vi "etlWriteFuncGenWithDelayedSignal.vi"(1 "max (dpt)":dbl, 2 "min (dpt)":dbl, 3 "minmax":bool) -> ()   [LabVIEW 2017]
uses:
  <vilib>/DAQmx/write.llb/DAQmx Write (Analog 2D DBL NChan NSamp).vi
  globalDevices.vi
  globalUtilities.vi
  <vilib>/DAQmx/miscellaneous.llb/DAQmx Fill In Error Info.vi
panel:
  out "max step":dbl
  out "success":bool
  out "Waveform Graph 3":dbl[][](graph)
  out "nT":i32
  out "dt":dbl
  out "omega":dbl
  out "amplitude":dbl
  out "offset":dbl
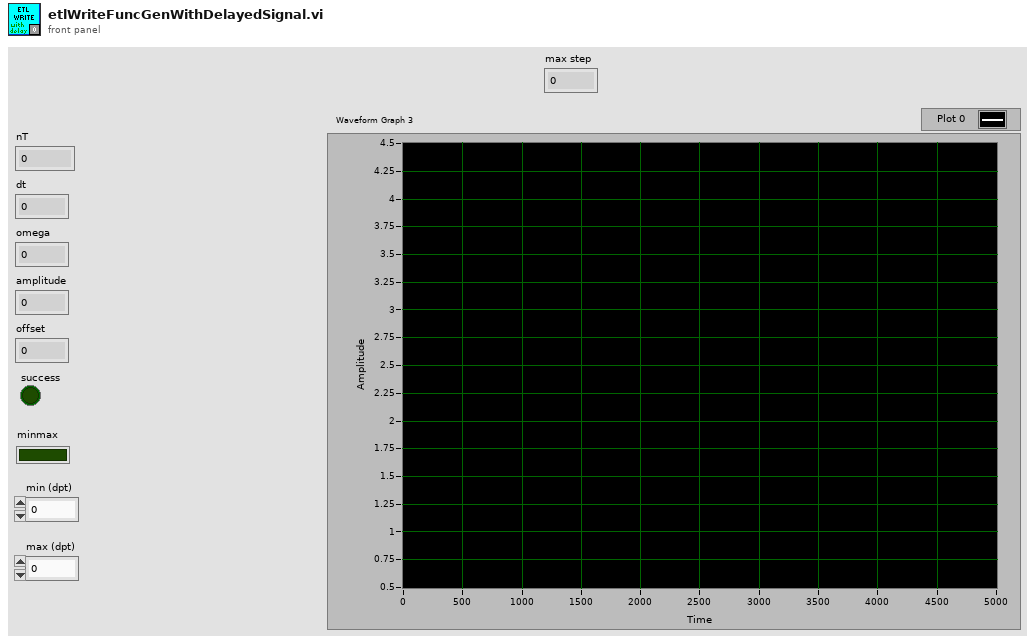
[diagram p1: front panel]
types:
  T1 = cluster{"waveform":dbl[], "latencyShiftPermutation":i32, "V/um":dbl, "waveType":string, "etlCalibrationMindpt":dbl, "etlCalibrationMaxdpt":dbl, "piezoEtlClockLock":bool, "volumeHeight":dbl, "volumeHeightUnits":string, "etl dpt/um":dbl, "etlVMin":dbl, "etlVMax":dbl}
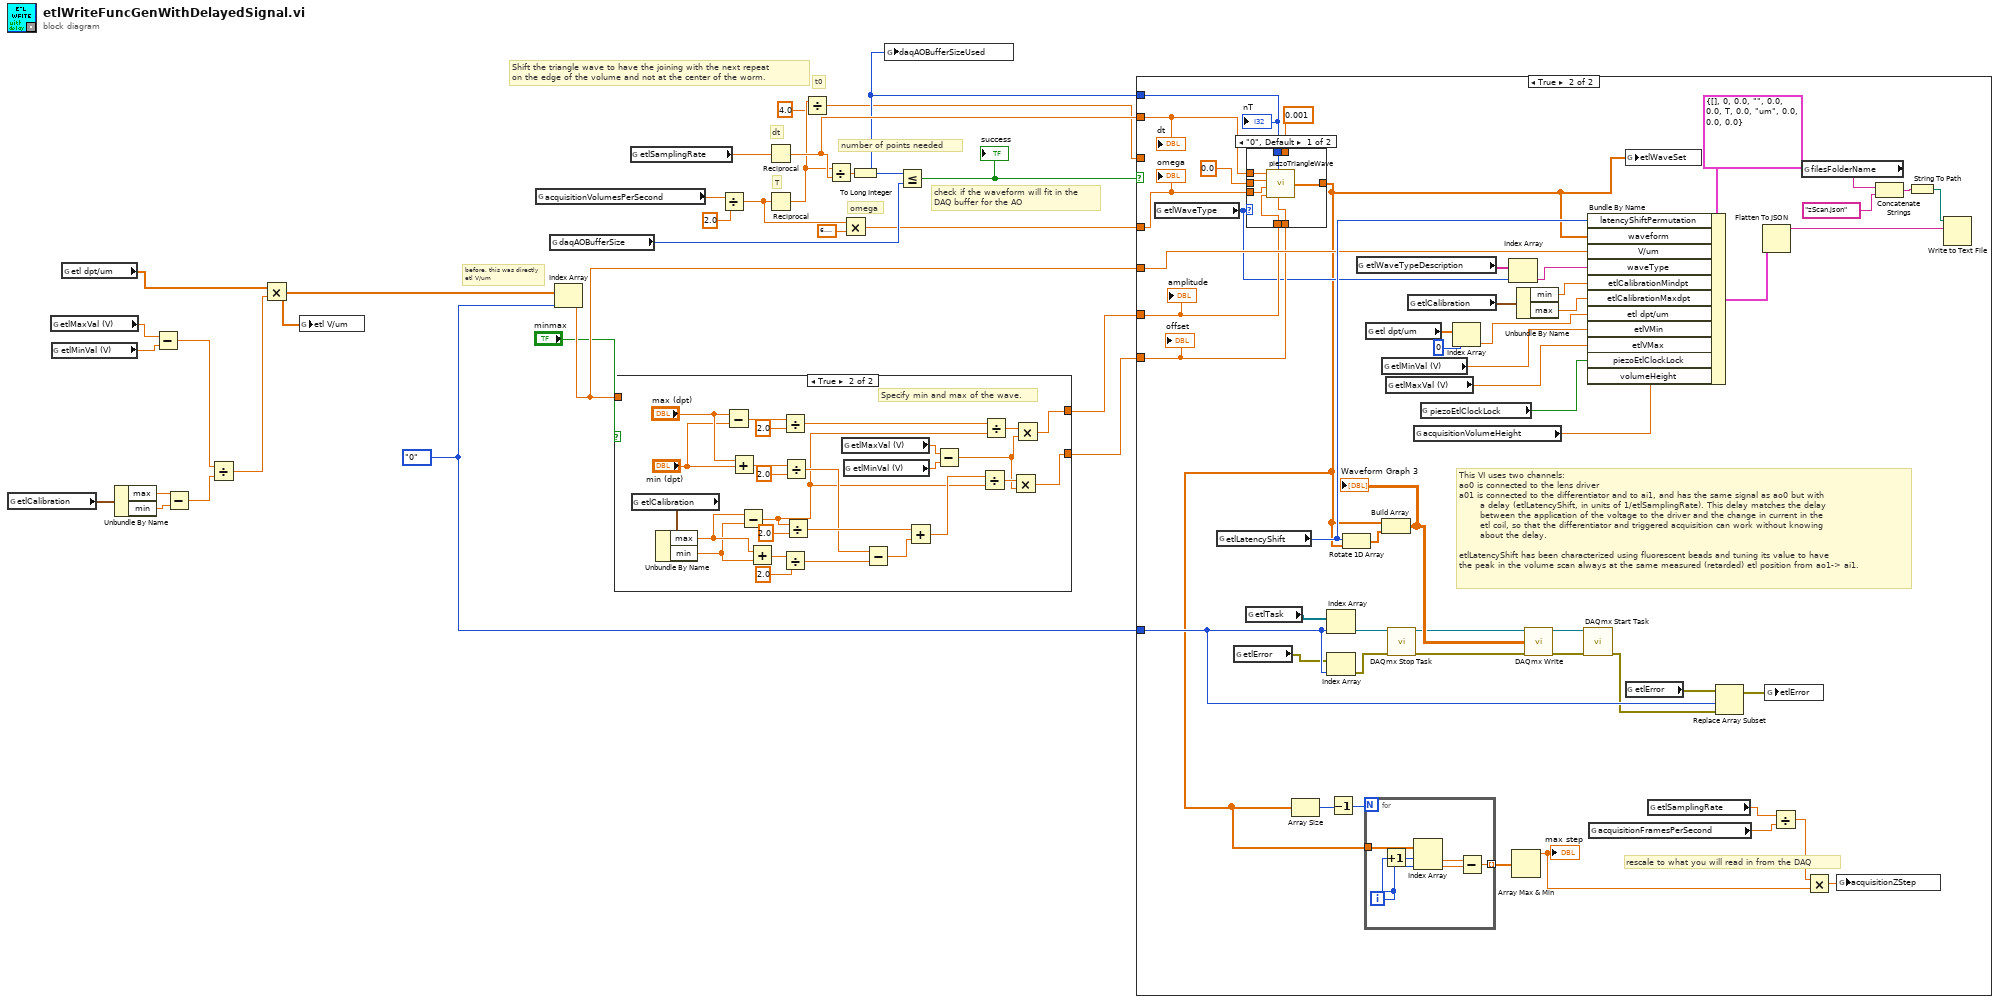
[diagram p0: block diagram]
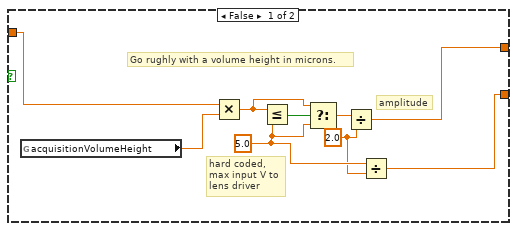
[diagram p2: hidden frame]
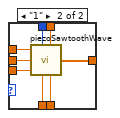
[diagram p4: hidden frame]
diagram:
  w17 = enum16{"0", "1"}."0" ("lens")
  # "Shift the triangle wave to have the joining with the next repeat\non the edge of the volume and not at the center of the worm."
  # "t0"
  # "before, this was directly\netl V/um"
  # "check if the waveform will fit in the\nDAQ buffer for the AO"
  # "omega"
  # "number of points needed"
  # "T"
  # "dt"
  n1 = global read "globalDevices.vi" "etlCalibration"() -> (w14:cluster{"min":dbl, "max":dbl})
  n2 = global read "globalDevices.vi" "etlMaxVal (V)"() -> (w11:dbl)
  n3 = global read "globalDevices.vi" "etlMinVal (V)"() -> (w10:dbl)
  n4 = global read "globalDevices.vi" "etl dpt/um"() -> (w7:dbl[])
  n5 = Unbundle By Name(w14) -> ("max"=w13:dbl, "min"=w12:dbl)
  n6 = Subtract(x=w11, y=w10) -> (x-y=w9:dbl)
  n7 = Subtract(x=w13, y=w12) -> (x-y=w8:dbl)
  n8 = Divide(x=w9, y=w8) -> (x/y=w6:dbl)
  n9 = Multiply(x=w7, y=w6) -> (x*y=w5:dbl[])
  n10 = global write "globalDevices.vi" "etl V/um"(w5) -> ()
  n11 = global read "globalUtilities.vi" "acquisitionVolumesPerSecond"() -> (w28:dbl)
  n12 = global read "globalDevices.vi" "daqAOBufferSize"() -> (w26:i32)
  n13 = Index Array(array=w5, index=w17) -> (element=w16:dbl)
  n14 = case shown="True" "minmax" {
    tunnel: [w34 w51] -> w25
    tunnel: [w31 w39] -> w18
    tunnel: w16 -> [w30 _]
    frame False {
      w33 = 5.0 ("y")
      w32 = 2.0 ("y")
      # "Go rughly with a volume height in microns."
      # "hard coded,\nmax input V to\nlens driver"
      # "amplitude"
      n15 = global read "globalUtilities.vi" "acquisitionVolumeHeight"() -> (w38:dbl)
      n16 = Multiply(x=w30, y=w38) -> (x*y=w36:dbl)
      n17 = Less Or Equal?(x=w36, y=w33) -> (x <= y?=w37:bool)
      n18 = Select(t=w36, s=w37, f=w33) -> (s? t:f=w35:dbl)
      n19 = Divide(x=w35, y=w32) -> (x/y=w34:dbl)
      n20 = Divide(x=w33, y=w32) -> (x/y=w31:dbl)
    }
    frame True {
      # "Specify min and max of the wave."
      n21 = global read "globalDevices.vi" "etlCalibration"() -> (w58:cluster{"min":dbl, "max":dbl})
      n22 = Unbundle By Name(w58) -> ("max"=w57:dbl, "min"=w56:dbl)
      n23 = Subtract(x="max (dpt)", y="min (dpt)") -> (x-y=w64:dbl)
      n24 = Add(x="max (dpt)", y="min (dpt)") -> (x+y=w59:dbl)
      n25 = Subtract(x=w57, y=w56) -> (x-y=w40:dbl)
      n26 = Add(x=w57, y=w56) -> (x+y=w55:dbl)
      n27 = Divide(x=w64, y=2.0) -> (x/y=w53:dbl)
      n28 = Divide(x=w55, y=2.0) -> (x/y=w47:dbl)
      n29 = Divide(x=w59, y=2.0) -> (x/y=w48:dbl)
      n30 = Divide(x=w40, y=2.0) -> (x/y=w49:dbl)
      n31 = global read "globalDevices.vi" "etlMaxVal (V)"() -> (w45:dbl)
      n32 = global read "globalDevices.vi" "etlMinVal (V)"() -> (w44:dbl)
      n33 = Subtract(x=w48, y=w47) -> (x-y=w46:dbl)
      n34 = Add(x=w49, y=w46) -> (x+y=w41:dbl)
      n35 = Subtract(x=w45, y=w44) -> (x-y=w42:dbl)
      n36 = Divide(x=w41, y=w40) -> (x/y=w43:dbl)
      n37 = Divide(x=w53, y=w40) -> (x/y=w52:dbl)
      n38 = Multiply(x=w43, y=w42) -> (x*y=w39:dbl)
      n39 = Multiply(x=w52, y=w42) -> (x*y=w51:dbl)
    }
  }
  n40 = global read "globalDevices.vi" "etlSamplingRate"() -> (w29:dbl)
  n41 = Divide(x=w28, y=2.0) -> (x/y=w23:dbl)
  n42 = Reciprocal(x=w29) -> (1/x=w21:dbl)
  n43 = Reciprocal(x=w23) -> (1/x=w3:dbl)
  n44 = Divide(x=w3, y=4.0) -> (x/y=w1:dbl)
  n45 = Divide(x=w3, y=w21) -> (x/y=w20:dbl)
  n46 = Multiply(x=w23, y=6.283185307179586) -> (x*y=w22:dbl)
  n47 = To Long Integer(number=w20) -> (32bit integer=w19:i32)
  n48 = global write "globalDevices.vi" "daqAOBufferSizeUsed"(w19) -> ()
  n49 = Less Or Equal?(x=w19, y=w26) -> (x <= y?=w4:bool)
  "success" <- w4
  n50 = case shown="True" w4 {
    tunnel: w25 -> [_ w109]
    tunnel: w18 -> [_ w110]
    tunnel: w22 -> [_ w108]
    tunnel: w19 -> [_ w106]
    tunnel: w21 -> [_ w107]
    tunnel: w17 -> [_ w116]
    tunnel: w16 -> [_ w111]
    tunnel: w1 -> [_ _]
    frame False {
    }
    frame True {
      # "rescale to what you will read in from the DAQ"
      # "This VI uses two channels:\nao0 is connected to the lens driver\na01 is connected to the differentiator and to ai1, and has the same signal as ao0 but with\n       a delay (etlLatencyShift, in units of 1/etlSamplingRate). This delay matches the delay \n       between the application of the voltage to the driver and the change in current in the\n       etl coil, so that the differentiator and triggered acquisition can work without knowing\n       about the delay.\n\netlLatencyShift has been characterized using fluorescent beads and tuning its value to have\nthe peak in the volume scan always at the same measured (retarded) etl position from ao1-> ai1."
      n51 = global read "globalDevices.vi" "etlWaveType"() -> (w102:enum16{"0", "1"})
      n52 = global read "globalDevices.vi" "etlLatencyShift"() -> (w115:i16)
      n53 = global read "globalDevices.vi" "etlError"() -> (w79:errorcluster[])
      n54 = global read "globalDevices.vi" "etlTask"() -> (w80:refnum<k21>[])
      n55 = case shown="\"0\", Default" w102 {
        tunnel: w110 -> [w124 w137]
        tunnel: w109 -> [w125 w136]
        tunnel: w108 -> [w126 w135]
        tunnel: 0.0 -> [w127 w134]
        tunnel: w107 -> [w128 w133]
        tunnel: w106 -> [w129 w132]
        tunnel: [w123 w131] -> w71
        tunnel: 0.001 ("smoothing param") -> [_ w130]
        frame "0", Default {
          n56 = call "piezoTriangleWave.vi"("offset"=w124, "nT"=w129, "amplitude"=w125, "omega"=w126, "t0"=w127, "dt"=w128) -> ("x+y"=w123:dbl[])
        }
        frame "1" {
          n57 = call "piezoSawtoothWave.vi"("dt"=w133, "nT"=w132, "t0"=w134, "omega"=w135, "amplitude"=w136, "smoothing param"=w130, "offset"=w137) -> ("x+y"=w131:dbl[])  [unwired: 2 in]
        }
      }
      n58 = Array Size(array=w71) -> (size(s)=w73:i32)
      n59 = Index Array(array=w80, index=w116) -> (element=w78:refnum<k21>)
      n60 = Index Array(array=w79, index=w116) -> (element=w77:errorcluster)
      n61 = Decrement(x=w73) -> (x-1=w72:i32)
      n62 = Rotate 1D Array(1:w71, 2:w115) -> (0:w98:dbl[])
      n63 = global read "globalDevices.vi" "etlWaveTypeDescription"() -> (w104:string[])
      n64 = for {
        N: w72 -> [_]
        tunnel: w71 -> [w122]
        tunnel: [w117] -> w70 mode=indexing
        i -> [w121]
        n65 = Increment(x=w121) -> (x+1=w120:i32)
        n66 = Index Array(array=w122, index #1=w120, index #2=w121) -> (element #1=w118:dbl, element #2=w119:dbl)
        n67 = Subtract(x=w118, y=w119) -> (x-y=w117:dbl)
      }
      n68 = global read "globalDevices.vi" "etl dpt/um"() -> (w90:dbl[])
      n69 = global read "globalDevices.vi" "etlMinVal (V)"() -> (w87:dbl)
      n70 = Build Array(w71, w98) -> (w97:dbl[][])
      "Waveform Graph 3" <- w97
      n71 = global read "globalDevices.vi" "etlMaxVal (V)"() -> (w86:dbl)
      n72 = call <vilib>:"DAQmx Stop Task.vi"("task/channels in"=w78, "error in"=w77) -> ("task out"=w81:refnum<k21>, "error out"=w82:errorcluster)  [unwired: 12 in]
      n73 = global read "globalDevices.vi" "etlCalibration"() -> (w101:cluster{"min":dbl, "max":dbl})
      n74 = global read "globalUtilities.vi" "acquisitionVolumeHeight"() -> (w92:dbl)
      n75 = global read "globalUtilities.vi" "piezoEtlClockLock"() -> (w91:bool)
      n76 = Index Array(array=w90, index=0) -> (element=w88:dbl)
      n77 = Index Array(array=w104, index=w102) -> (element=w103:string)
      n78 = Array Max & Min(array=w70) -> (max value=w65:dbl)  [unwired: 3 out]
      "max step" <- w65
      n79 = Unbundle By Name(w101) -> ("min"=w100:dbl, "max"=w99:dbl)
      n80 = call-poly <vilib>:"DAQmx Write.vi"("task/channels in"=w81, "data"=w97, "error in"=w82) -> ("task out"=w83:refnum<k21>, "error out"=w84:errorcluster)  [unwired: 10 in, 1 out]
      n81 = call <vilib>:"DAQmx Start Task.vi"("task/channels in"=w83, "error in"=w84) -> ("error out"=w75:errorcluster)  [unwired: 12 in, 1 out]
      n82 = Bundle By Name(cluster=T1 {"waveform"=[], "latencyShiftPermutation"=0, "V/um"=0.0, "waveType"="", "etlCalibrationMindpt"=0.0, "etlCalibrationMaxdpt"=0.0, "piezoEtlClockLock"=TRUE, "volumeHeight"=0.0, "volumeHeightUnits"="um", "etl dpt/um"=0.0, "etlVMin"=0.0, "etlVMax"=0.0} ("input cluster"), "latencyShiftPermutation"=w115, "waveform"=w71, "V/um"=w111, "waveType"=w103, "etlCalibrationMindpt"=w100, "etlCalibrationMaxdpt"=w99, "etl dpt/um"=w88, "etlVMin"=w87, "etlVMax"=w86, "piezoEtlClockLock"=w91, "volumeHeight"=w92) -> (w113:T1)
      n83 = global read "globalUtilities.vi" "acquisitionFramesPerSecond"() -> (w68:dbl)
      n84 = global write "globalDevices.vi" "etlWaveSet"(w71) -> ()
      n85 = global read "globalDevices.vi" "etlError"() -> (w76:errorcluster[])
      n86 = global read "globalDevices.vi" "etlSamplingRate"() -> (w69:dbl)
      n87 = Replace Array Subset(array=w76, new element=w75, index=w116) -> (w74:errorcluster[])
      n88 = Flatten To JSON(anything=w113) -> (JSON string=w112:string)  [unwired: 2 in, 1 out]
      n89 = global write "globalDevices.vi" "etlError"(w74) -> ()
      n90 = Divide(x=w69, y=w68) -> (x/y=w66:dbl)
      n91 = global read "globalUtilities.vi" "filesFolderName"() -> (w96:string)
      n92 = Multiply(x=w66, y=w65) -> (x*y=w67:dbl)
      n93 = global write "globalUtilities.vi" "acquisitionZStep"(w67) -> ()
      n94 = Concatenate Strings(w96, "zScan.json" ("string")) -> (w94:string)
      n95 = String To Path(string=w94) -> (path=w93:path)
      n96 = Write to Text File(file (use dialog)=w93, text=w112) -> ()  [unwired: 2 in, 3 out]
      "nT" <- w106
      "dt" <- w107
      "omega" <- w108
      "amplitude" <- w109
      "offset" <- w110
    }
  }
